vi "GantryGlobals.vi"() -> ()   [LabVIEW 2014]
panel:
  out "LiftSetTripped":bool
  out "RobotMoving":bool
  out "RobotAligned":bool
  out "NudgeEnabled":bool
  in  "LiftError":dbl
  in  "ArmError":dbl
  in  "GantryError":dbl
  in  "ArmSetpoint":dbl
  in  "GantrySetpoint":dbl
  in  "LiftSetpoint":dbl
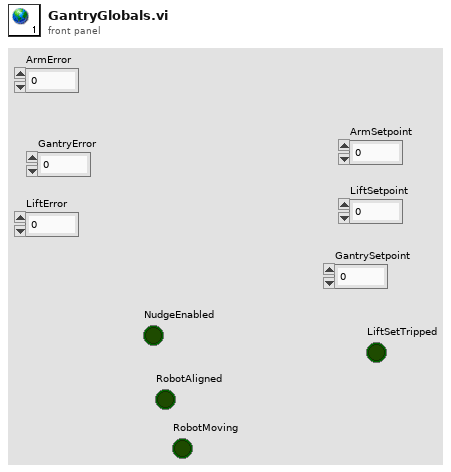
[diagram p1: front panel]
diagram:
